vi "SwitchTillOn.vi"(5 "Stop if On?":bool, 7 "Turn Off Button":refnum<vi>, 9 "timeout":u32, 10 "Turn On Button":refnum<vi>, 11 "Turn On Indicator":refnum<vi>) -> (3 "Success?":bool)   [LabVIEW 2020]
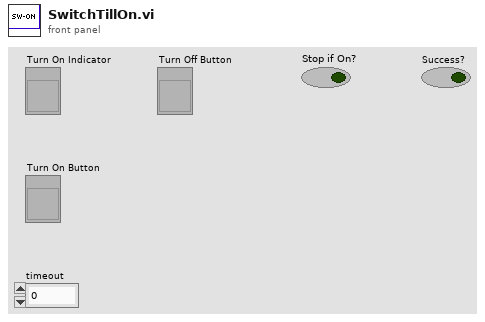
[diagram p1: front panel]
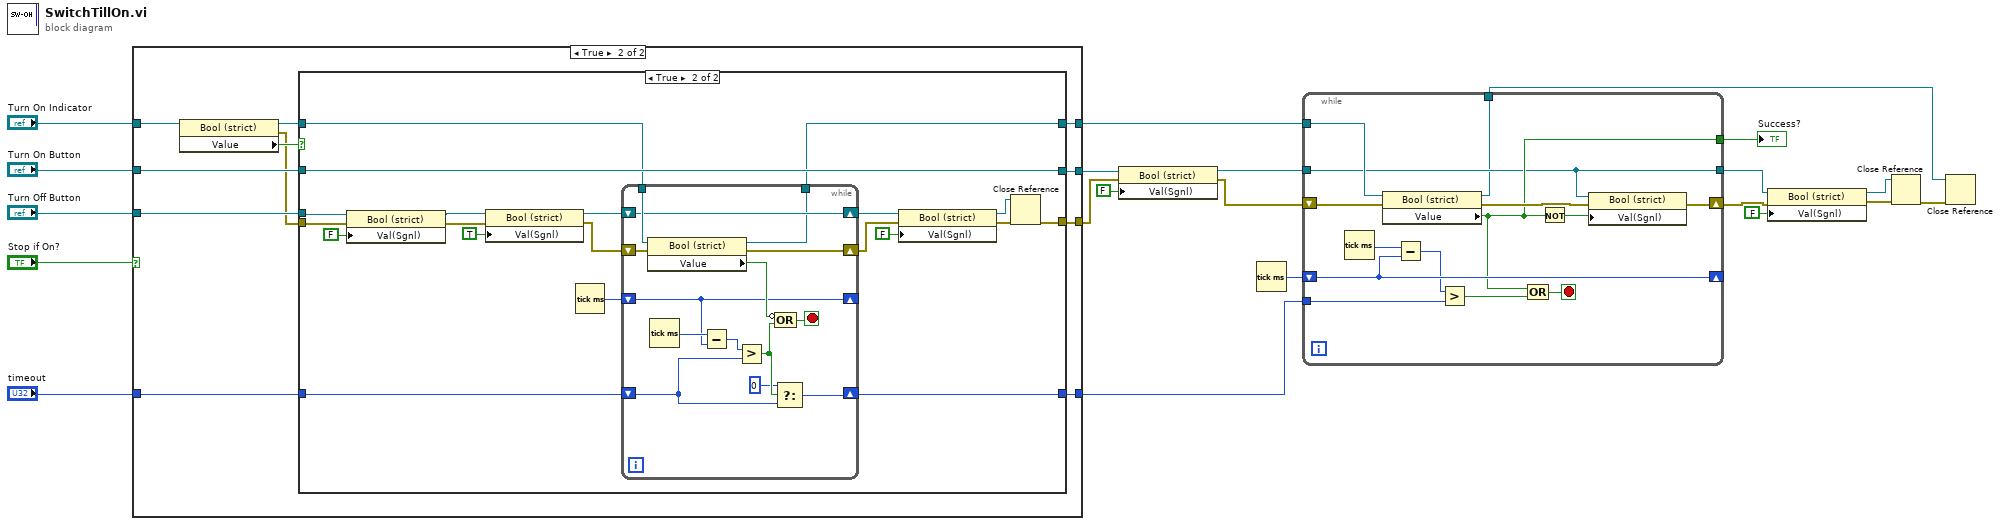
[diagram p0: block diagram]
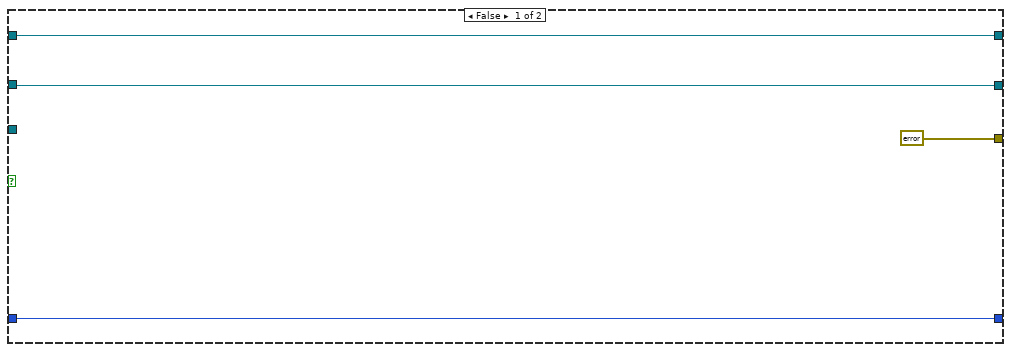
[diagram p2: hidden frame]
diagram:
  n1 = case shown="True" "Stop if On?" {
    tunnel: "Turn On Indicator" -> [w25 w36]
    tunnel: [w25 w33] -> w16
    tunnel: "Turn On Button" -> [w24 w32]
    tunnel: [w24 w31] -> w14
    tunnel: "Turn Off Button" -> [_ w30]
    tunnel: "timeout" -> [w23 w29]
    tunnel: [w23 w28] -> w10
    tunnel: [errorcluster {"status"=FALSE, "code"=0, "source"=""} ("error out") w26] -> w6
    frame False {
    }
    frame True {
      n2 = property class="Bool (strict)"(reference=w36) -> (reference out=w34:refnum<vi>, error out=w27:errorcluster, "Value"=w35:bool)  [unwired: 1 in]
      n3 = case shown="True" w35 {
        tunnel: w34 -> [w40 w44]
        tunnel: [w40 w45] -> w33
        tunnel: w32 -> [w39 w60]
        tunnel: [w39 w60] -> w31
        tunnel: w30 -> [_ w50]
        tunnel: w29 -> [w38 w56]
        tunnel: [w38 w53] -> w28
        tunnel: w27 -> [w37 w49]
        tunnel: [w37 w42] -> w26
        frame False {
        }
        frame True {
          n4 = property class="Bool (strict)"(reference=w50, error in=w49, "Val(Sgnl)"=FALSE ("Value (Signaling)")) -> (reference out=w51:refnum<vi>, error out=w48:errorcluster)
          n5 = property class="Bool (strict)"(reference=w51, error in=w48, "Val(Sgnl)"=TRUE ("Value (Signaling)")) -> (reference out=w58:refnum<vi>, error out=w47:errorcluster)
          n6 = Tick Count (ms)() -> (millisecond timer value=w57:u32)
          n7 = while {
            tunnel: w44 -> [w73]
            shift-right: [w71] -> _
            shift-left: w57 -> [w71]
            shift-right: [w68] -> w54
            shift-left: w58 -> [w68]
            shift-right: [w66] -> w53
            shift-left: w56 -> [w67]
            shift-right: [w62] -> w46
            shift-left: w47 -> [w63]
            tunnel: [w61] -> w45
            stop <- w69 stop-if-true
            n8 = property class="Bool (strict)"(reference=w73, error in=w63) -> (reference out=w61:refnum<vi>, error out=w62:errorcluster, "Value"=w74:bool)
            n9 = Tick Count (ms)() -> (millisecond timer value=w72:u32)
            n10 = Subtract(x=w72, y=w71) -> (x-y=w70:u32)
            n11 = Greater?(x=w70, y=w67) -> (0:w65:bool)
            n12 = Compound Arithmetic op=OR(invert w74, w65) -> (w69:bool)
            n13 = Select(t=u32 0, s=w65, f=w67) -> (s? t:f=w66:u32)
          }
          n14 = property class="Bool (strict)"(reference=w54, error in=w46, "Val(Sgnl)"=FALSE ("Value (Signaling)")) -> (reference out=w41:refnum<vi>, error out=w43:errorcluster)
          n15 = Close Reference(reference=w41, error in (no error)=w43) -> (error out=w42:errorcluster)
        }
      }
    }
  }
  n16 = property class="Bool (strict)"(reference=w14, error in=w6, "Val(Sgnl)"=FALSE ("Value (Signaling)")) -> (reference out=w18:refnum<vi>, error out=w5:errorcluster)
  n17 = Tick Count (ms)() -> (millisecond timer value=w20:u32)
  n18 = while {
    tunnel: w18 -> [w76]
    shift-right: [w88] -> w7
    shift-left: w5 -> [w86]
    tunnel: w16 -> [w84]
    shift-right: [w82] -> _
    shift-left: w20 -> [w82]
    tunnel: w10 -> [w80]
    tunnel: [w77] -> w21
    tunnel: [w76] -> w8
    tunnel: [w75] -> w2
    stop <- w79 stop-if-true
    n19 = Tick Count (ms)() -> (millisecond timer value=w83:u32)
    n20 = property class="Bool (strict)"(reference=w84, error in=w86) -> (reference out=w75:refnum<vi>, error out=w85:errorcluster, "Value"=w77:bool)
    n21 = Subtract(x=w83, y=w82) -> (x-y=w81:u32)
    n22 = Greater?(x=w81, y=w80) -> (0:w78:bool)
    n23 = Or(x=w77, y=w78) -> (x .or. y?=w79:bool)
    n24 = Not(x=w77) -> (.not. x?=w87:bool)
    n25 = property class="Bool (strict)"(reference=w76, error in=w85, "Val(Sgnl)"=w87) -> (error out=w88:errorcluster)  [unwired: 1 out]
  }
  "Success?" <- w21
  n26 = property class="Bool (strict)"(reference=w8, error in=w7, "Val(Sgnl)"=FALSE ("Value (Signaling)")) -> (reference out=w3:refnum<vi>, error out=w4:errorcluster)
  n27 = Close Reference(reference=w3, error in (no error)=w4) -> (error out=w1:errorcluster)
  n28 = Close Reference(reference=w2, error in (no error)=w1) -> ()  [unwired: 1 out]
